vi "XY Chart Buffer V5.vi"(8 "Clear History? (default: no)":bool, 9 "History Length (default:1000)":i32=1000, 10 "New Point":cluster{"x":dbl, "y":dbl} {"y" format="%.2f"; "x" format="%.2f"}, 11 "New Points":cluster{"x":dbl, "y":dbl}[](array[cluster]) {"y" format="%.2f"; "x" format="%.2f"}) -> (3 "XY Chart Data":cluster{"x":dbl, "y":dbl}[](array[cluster]) {"y" format="%.2f"; "x" format="%.2f"})   [LabVIEW 2013]
doc: "This reentrant VI uses an XY graph to mimic the behavior of an XY chart, in that it plots a stipulated amount of the most recently acquired data points. The chart data is stored in a static local variable of the output XY chart indicator.\n\nBecause the VI has been marked reentrant (in VI setup), you can make multiple parallel calls to the VI without confusing the memory. Use the new points array input to supply multiple points at once, or leave the array unwired (empty) and use the new point cluster input to supply one point at a time. If the locally stored chart array is not equal to chart length, it is expanded to that lenght by replicating the most recently acquired point. Data in excess of the history length is discarded. Set clear first to clear the chart history before processing the new points."
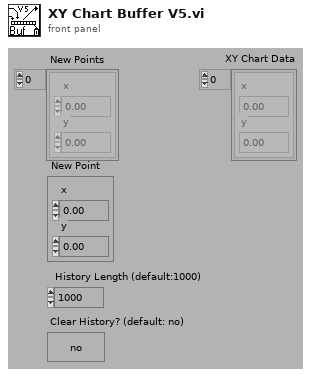
[diagram p1: front panel]
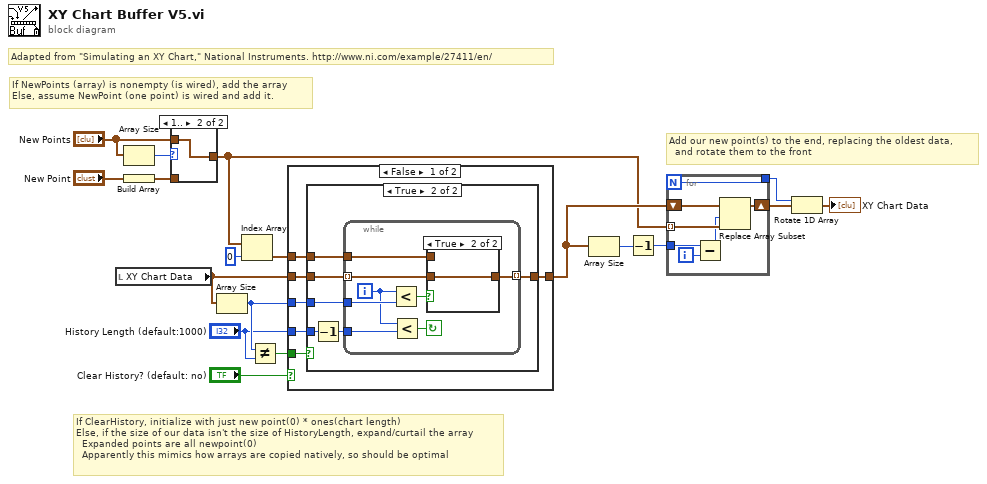
[diagram p0: block diagram]
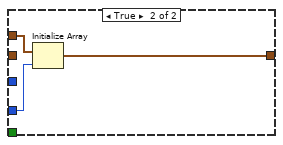
[diagram p4: hidden frame]
diagram:
  # "Add our new point(s) to the end, replacing the oldest data,\n  and rotate them to the front"
  # "If ClearHistory, initialize with just new point(0) * ones(chart length)\nElse, if the size of our data isn't the size of HistoryLength, expand/curtail the array\n  Expanded points are all newpoint(0)\n  Apparently this mimics how arrays are copied natively, so should be optimal"
  # "If NewPoints (array) is nonempty (is wired), add the array\nElse, assume NewPoint (one point) is wired and add it."
  # "Adapted from \"Simulating an XY Chart,\" National Instruments. http://www.ni.com/example/27411/en/"
  n1 = local read "XY Chart Data"() -> (w12:cluster{"x":dbl, "y":dbl}[])
  n2 = Array Size(array="New Points") -> (size(s)=w16:i32)
  n3 = Build Array("New Point") -> (w18:cluster{"x":dbl, "y":dbl}[])
  n4 = case shown="1.." w16 {
    tunnel: [w19 w20] -> w6
    tunnel: "New Points" -> [_ w20]
    tunnel: w18 -> [w19 _]
    frame ..0 {
    }
    frame 1.. {
    }
  }
  n5 = Array Size(array=w12) -> (size(s)=w11:i32)
  n6 = Index Array(array=w6, index=0) -> (element=w5:cluster{"x":dbl, "y":dbl})
  n7 = Not Equal?(x=w11, y="History Length (default:1000)") -> (x != y?=w4:bool)
  n8 = case shown="False" "Clear History? (default: no)" {
    tunnel: w4 -> [w26 _]
    tunnel: "History Length (default:1000)" -> [w25 w45]
    tunnel: w12 -> [w24 _]
    tunnel: w11 -> [w23 _]
    tunnel: w5 -> [w22 w46]
    tunnel: [w21 w44] -> w9
    frame False {
      n9 = case shown="True" w26 {
        tunnel: [w27 w31] -> w21
        tunnel: w25 -> [_ w32]
        tunnel: w24 -> [w27 w33]
        tunnel: w22 -> [_ w29]
        tunnel: w23 -> [_ w30]
        frame False {
        }
        frame True {
          n10 = Decrement(x=w32) -> (x-1=w28:i32)
          n11 = while {
            tunnel: [w40] -> w31 mode=indexing
            tunnel: w29 -> [w38]
            tunnel: w28 -> [w34]
            tunnel: w33 -> [w39] mode=indexing
            tunnel: w30 -> [w37]
            i -> [w36]
            stop <- w41 continue-if-true
            n12 = Less?(x=w36, y=w37) -> (x < y?=w35:bool)
            n13 = Less?(x=w36, y=w34) -> (x < y?=w41:bool)
            n14 = case shown="True" w35 {
              tunnel: [w42 w43] -> w40
              tunnel: w39 -> [_ w43]
              tunnel: w38 -> [w42 _]
              frame False {
              }
              frame True {
              }
            }
          }
        }
      }
    }
    frame True {
      n15 = Initialize Array(w46, w45) -> (w44:cluster{"x":dbl, "y":dbl}[])
    }
  }
  n16 = Array Size(array=w9) -> (size(s)=w3:i32)
  n17 = Decrement(x=w3) -> (x-1=w2:i32)
  n18 = for {
    N -> [w48]
    shift-right: [w53] -> w14
    shift-left: w9 -> [w51]
    tunnel: w6 -> [w52] mode=indexing
    tunnel: [w48] -> w10
    tunnel: w2 -> [w47]
    i -> [w49]
    n19 = Subtract(x=w47, y=w49) -> (x-y=w50:i32)
    n20 = Replace Array Subset(array=w51, new element=w52, index=w50) -> (w53:cluster{"x":dbl, "y":dbl}[])
  }
  n21 = Rotate 1D Array(1:w14, 2:w10) -> (0:→"XY Chart Data":cluster{"x":dbl, "y":dbl}[])
